vi "gen MB frame -Set the Baudrate.vi"(9 "baudrate":T1=3 items=["4800"=2, "9600"=3, "19200"=4], 11 "Dev Addr":u8=1 format="%x") -> (3 "MB frame":string)   [LabVIEW 2016, in "MB _relays.lvlib"]
uses:
  MB _relays.lvlib
  type defs/baudrate.ctl
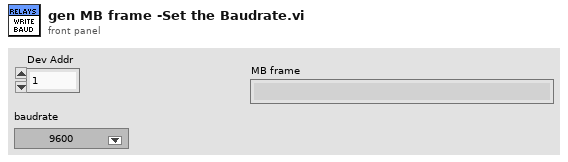
[diagram p1: front panel]
types:
  T1 = typedef "MB _relays.lvlib/baudrate.ctl" = u8
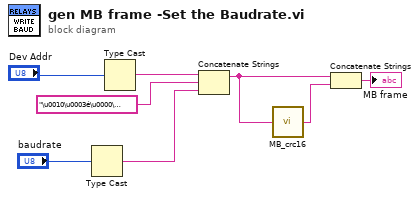
[diagram p0: block diagram]
diagram:
  n1 = Type Cast(x="baudrate") -> (*(type *) &x=w1:string)  [unwired: 1 in]
  n2 = Type Cast(x="Dev Addr") -> (*(type *) &x=w7:string)  [unwired: 1 in]
  n3 = Concatenate Strings(w7, "\u0010\u0003é\u0000\u0001\u0002\u0000", w1) -> (w5:string)
  n4 = call "MB_crc16.vi"("message"=w5) -> ("CRC16"=w4:string)  [unwired: 4 in]
  n5 = Concatenate Strings(w5, w4) -> (→"MB frame":string)
